vi "Reset Message Class.vi"(8 "error in (no error)":errorcluster, 9 "Template Path":path, 10 "Message Class":refnum<vi>) -> (0 "error out":errorcluster)   [LabVIEW 2023, in "Message Maker.lvclass"]
doc: "Clears the front panle and block diagram of the Do and Send methods and preps them to be modifed by the message maker code\n\nAuthor: Derek Trepanier\nCopyright: MGI 2015"
uses:
  Message Maker.lvclass
  Message Maker.lvclass/Message Maker.ctl
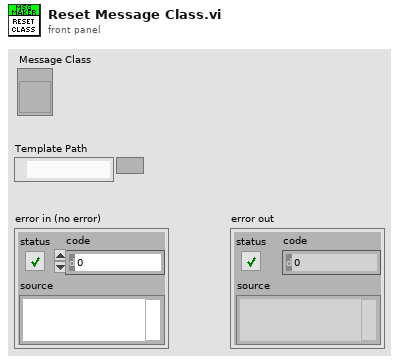
[diagram p1: front panel]
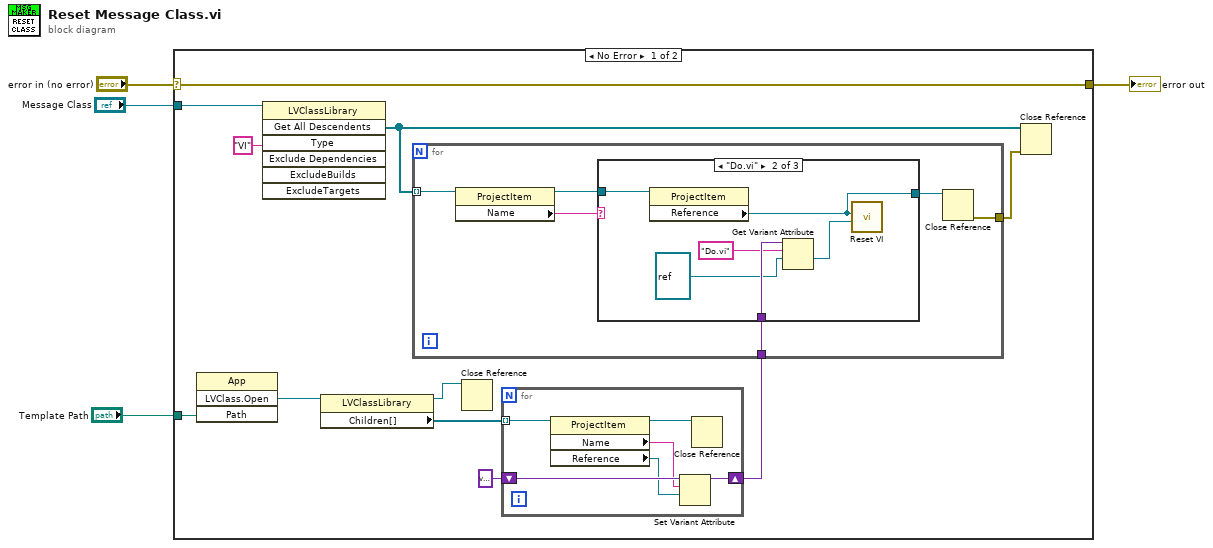
[diagram p0: block diagram]
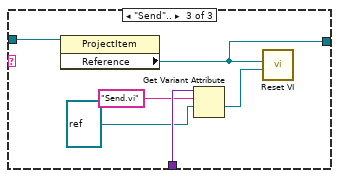
[diagram p3: hidden frame]
diagram:
  n1 = case shown="No Error" "error in (no error)" {
    selector: "error in (no error)" -> [w5 w40]
    tunnel: "Message Class" -> [w8 _]
    tunnel: "Template Path" -> [w7 _]
    tunnel: [w5 w40] -> w1
    frame No Error {
      n2 = invoke class="App" method="LVClass.Open"("Path"=w7) -> ("LVClass.Open"=w6:refnum<vi>)  [unwired: 3 in, 3 out]
      n3 = invoke class="LVClassLibrary" method="Get All Descendents"(reference=w8, "Type"="VI") -> ("All Descendents"=w14:refnum<vi>[])  [unwired: 5 in, 6 out]
      n4 = property class="LVClassLibrary"(reference=w6) -> (reference out=w13:refnum<vi>, "Children[]"=w10:refnum<vi>[])  [unwired: 1 in, 1 out]
      n5 = Close Reference(reference=w13) -> ()  [unwired: 1 in, 1 out]
      n6 = for {
        tunnel: w10 -> [w21] mode=indexing
        shift-right: [w20] -> w12
        shift-left: variant -> [w19]
        n7 = property class="ProjectItem"(reference=w21) -> (reference out=w16:refnum<vi>, "Name"=w18:string, "Reference"=w17:refnum<vi>)  [unwired: 1 in, 1 out]
        n8 = Set Variant Attribute(Variant=w19, name=w18, value=w17) -> (Variant out=w20:variant)  [unwired: 1 in, 2 out]
        n9 = Close Reference(reference=w16) -> ()  [unwired: 1 in, 1 out]
      }
      n10 = for {
        tunnel: w14 -> [w27] mode=indexing
        tunnel: w12 -> [w25]
        tunnel: [w22] -> w15
        n11 = property class="ProjectItem"(reference=w27) -> (reference out=w24:refnum<vi>, "Name"=w26:string)  [unwired: 1 in, 1 out]
        n12 = case shown="\"Do.vi\"" w26 {
          tunnel: w25 -> [_ w33 w39]
          tunnel: w24 -> [_ w30 w36]
          tunnel: [_ w28 w34] -> w23
          frame Default {
          }
          frame "Do.vi" {
            n13 = property class="ProjectItem"(reference=w30) -> ("Reference"=w28:refnum<vi>)  [unwired: 1 in, 2 out]
            n14 = Get Variant Attribute(Variant=w33, name="Do.vi", default value (empty Variant)=refnum<vi> refnum ("VI Reference")) -> (value=w29:refnum<vi>)  [unwired: 1 in, 3 out]
            n15 = call "Reset VI.vi"("Template"=w29, "Destination"=w28) -> ()  [unwired: 9 in, 1 out]
          }
          frame "Send".. {
            n16 = property class="ProjectItem"(reference=w36) -> ("Reference"=w34:refnum<vi>)  [unwired: 1 in, 2 out]
            n17 = Get Variant Attribute(Variant=w39, name="Send.vi", default value (empty Variant)=refnum<vi> refnum ("VI Reference")) -> (value=w35:refnum<vi>)  [unwired: 1 in, 3 out]
            n18 = call "Reset VI.vi"("Template"=w35, "Destination"=w34) -> ()  [unwired: 9 in, 1 out]
          }
        }
        n19 = Close Reference(reference=w23) -> (error out=w22:errorcluster)  [unwired: 1 in]
      }
      n20 = Close Reference(reference=w14, error in (no error)=w15) -> ()  [unwired: 1 out]
    }
    frame Error {
    }
  }
  "error out" <- w1
